vi "System Explorer - Add extra pages to System Explorer library.vi"(8 "error in (no error)":errorcluster, 9 "Extra Page Names":string[](array[string]), 10 "Project Root":path, 11 "ProjectItem in":refnum<vi>) -> (0 "error out":errorcluster, 3 "ProjectItem out":refnum<vi>)   [LabVIEW 2015, in "NIVS_Consolidated_CDW_MetaDataObj.lvclass"]
doc: "Create an addition folder under the ProjectItem and add all created extra pages to this folder."
uses:
  NIVS_Consolidated_CDW_MetaDataObj.lvclass
  CD System Explorer lvlib.ctl
  Add Item - Type.ctl
  CD System Explorer lvlib.vi
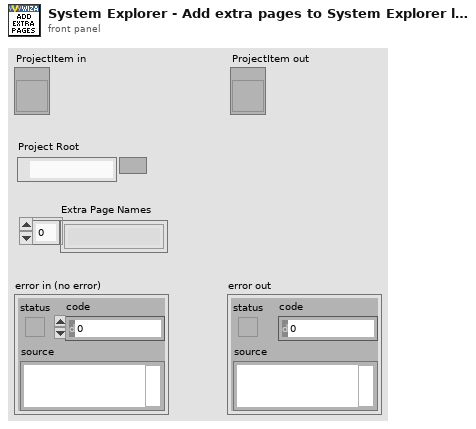
[diagram p1: front panel]
types:
  T1 = typedef "NIVS_Consolidated_CDW_MetaDataObj.lvclass/CD System Explorer lvlib.ctl" = enum16{"LibraryFileName", "LibraryFolderName", "System Explorer.FolderName", "System Explorer.Dynamically Called.FolderName", "System Explorer.Dynamically Called.Extra Pages.FolderName", "System Explorer.Dynamically Called.Extra Pages.TemplatePathAndName", "System Explorer.Dynamically Called.Main Page.VIName", "System Explorer.Dynamically Called.Main Page.TemplatePathAndName", "System Explorer.Dynamically Called.Initialization VI.VIName", "System Explorer.Dynamically Called.Initialization VI.TemplatePathAndName", "System Explorer.SubVI.FolderName", "System Explorer.Types.FolderName", "System Explorer.ActionVIOnCompile.VIName", "System Explorer.ExportConfigRTM.VIName", "System Explorer.LoadHelpFile.VIName"}
  T2 = typedef "NIVS_Consolidated_CDW_MetaDataObj.lvclass/Add Item - Type.ctl" = string
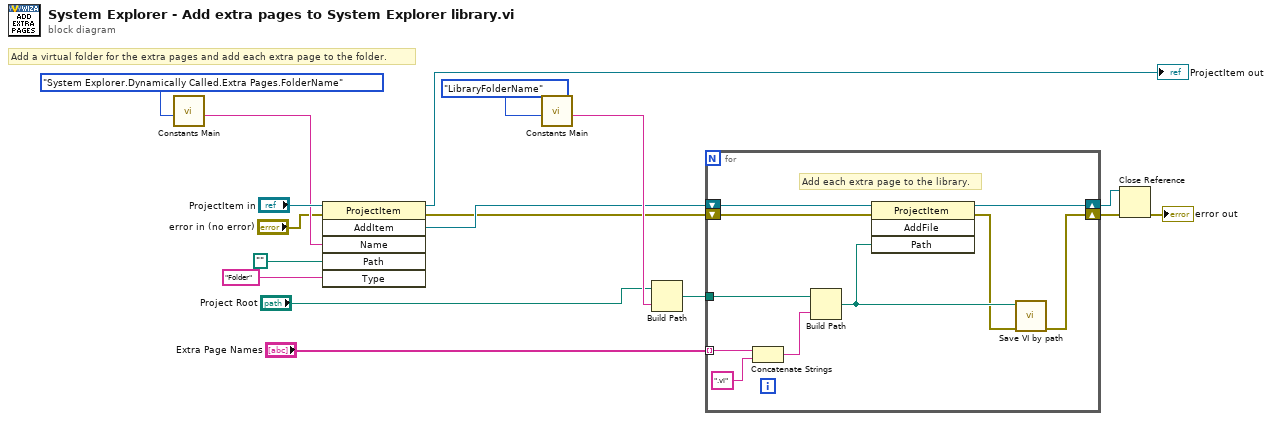
[diagram p0: block diagram]
diagram:
  # "Add a virtual folder for the extra pages and add each extra page to the folder."
  n1 = call-poly "Constants Main.vi"("Action"=CD_System_Explorer_lvlib."System Explorer.Dynamically Called.Extra Pages.FolderName") -> ("Output"=w12:string)  [unwired: 10 in]
  n2 = invoke class="ProjectItem" method="AddItem"(reference="ProjectItem in", error in="error in (no error)", "Name"=w12, "Path"=path "", "Type"=T2 "Folder" ("Add Item - Type")) -> (reference out=→"ProjectItem out":refnum<vi>, error out=w3:errorcluster, "AddItem"=w7:refnum<vi>)  [unwired: 1 in, 3 out]
  n3 = call-poly "Constants Main.vi"("Action"=CD_System_Explorer_lvlib."LibraryFolderName") -> ("Output"=w9:string)  [unwired: 10 in]
  n4 = Build Path(base path="Project Root", name or relative path=w9) -> (appended path=w8:path)
  n5 = for {
    shift-right: [w25] -> w5
    shift-left: w7 -> [w27]
    shift-right: [w19] -> w6
    shift-left: w3 -> [w26]
    tunnel: w8 -> [w22]
    tunnel: "Extra Page Names" -> [w18] mode=indexing
    # "Add each extra page to the library."
    n6 = Concatenate Strings(w18, ".vi") -> (w23:string)
    n7 = Build Path(base path=w22, name or relative path=w23) -> (appended path=w21:path)
    n8 = invoke class="ProjectItem" method="AddFile"(reference=w27, error in=w26, "Path"=w21) -> (reference out=w25:refnum<vi>, error out=w20:errorcluster)  [unwired: 1 in, 2 out]
    n9 = call "Save VI by path.vi"("error in (no error)"=w20, "VI path"=w21) -> ("error out"=w19:errorcluster)  [unwired: 9 in]
  }
  n10 = Close Reference(reference=w5, error in (no error)=w6) -> (error out=→"error out":errorcluster)
